vi "TX Message.vi"(8 "error in (no error)":errorcluster, 10 "variant":variant, 11 "Engine RPM in":refnum<class "Fuel Level Input.lvclass">) -> (0 "error out":errorcluster, 3 "Engine RPM out":refnum<class "Fuel Level Input.lvclass">)   [LabVIEW 2011, in "Fuel Level Input.lvclass"]
uses:
  Fuel Level Input.lvclass
  PID.lvclass
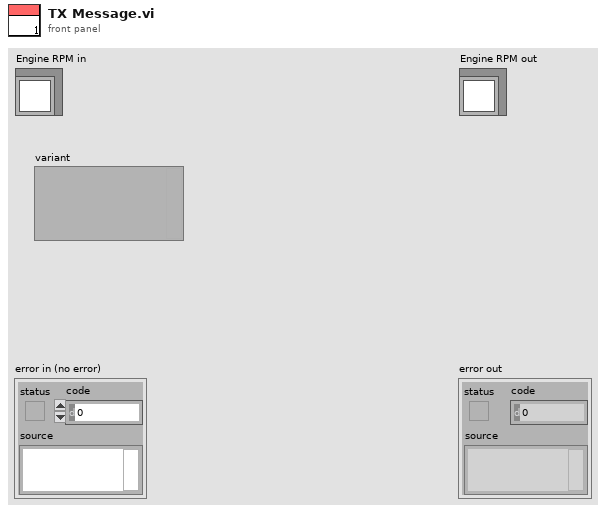
[diagram p1: front panel]
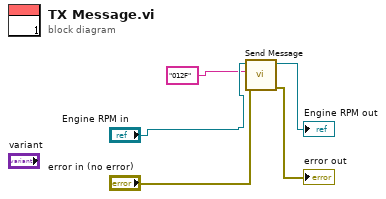
[diagram p0: block diagram]
diagram:
  n1 = call "Send Message.vi"("error in (no error)"="error in (no error)", "TX Message"="012F", "PID in"="Engine RPM in") -> ("error out"=→"error out":errorcluster, "PID out"=→"Engine RPM out":refnum<class "Fuel Level Input.lvclass">)  [unwired: 7 in]
